vi "decode_nanotech_read.vi"(9 "Data-Size (in Byte)":u8, 11 "read buffer in":string) -> (2 "Numeric Output":i32, 3 "read buffer out":string)   [LabVIEW 2021]
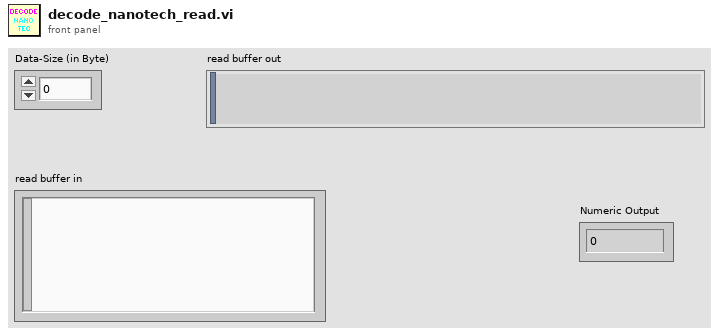
[diagram p1: front panel]
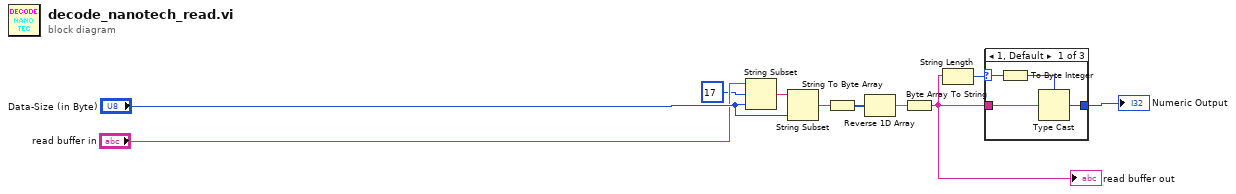
[diagram p0: block diagram]
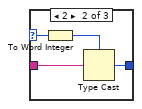
[diagram p2: hidden frame]
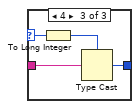
[diagram p3: hidden frame]
diagram:
  n1 = String Subset(string="read buffer in", offset (0)=u8 17 ("x"), length (rest)="Data-Size (in Byte)") -> (substring=w6:string)
  n2 = String Subset(string=w6, length (rest)="Data-Size (in Byte)") -> (substring=w3:string)  [unwired: 1 in]
  n3 = String To Byte Array(string=w3) -> (unsigned byte array=w4:u8[])
  n4 = Reverse 1D Array(array=w4) -> (reversed array=w5:u8[])
  n5 = Byte Array To String(unsigned byte array=w5) -> (string=w1:string)
  "read buffer out" <- w1
  n6 = String Length(string=w1) -> (length=w2:i32)
  n7 = case shown="1, Default" w2 {
    selector: w2 -> [w14 w18 w22]
    tunnel: w1 -> [w11 w16 w21]
    tunnel: [w12 w15 w20] -> w8
    frame 1, Default {
      n8 = To Byte Integer(number=w14) -> (8bit integer=w13:i8)
      n9 = Type Cast(type=w13, x=w11) -> (*(type *) &x=w12:i8)
    }
    frame 2 {
      n10 = To Word Integer(number=w18) -> (16bit integer=w17:i16)
      n11 = Type Cast(type=w17, x=w16) -> (*(type *) &x=w15:i16)
    }
    frame 4 {
      n12 = To Long Integer(number=w22) -> (32bit integer=w19:i32)
      n13 = Type Cast(type=w19, x=w21) -> (*(type *) &x=w20:i32)
    }
  }
  "Numeric Output" <- w8
